vi "burst_config.vi"(8 "error in (no error)":errorcluster, 11 "wf_multi":T1(array[cluster])=[{"device"="waveform_gen", "chan"=1}, {"device"="wf_33500B", "chan"=2}] {"chan" items=["1"=1, "2"=2]}) -> (0 "error out":errorcluster, 1 "cmds":string[](array[string])=["SOUR1:BURS:PHAS 0;\nSOUR1:BURS:MODE GAT;\nSOUR1:BURS:STAT ON;\nTRIG1:SLOP POS;\nTRIG1:DEL 0;\nTRIG1:SOUR EXT;", "SOUR1:BURS:PHAS 0;\nSOUR1:BURS:MODE GAT;\nSOUR1:BURS:STAT ON;\nTRIG1:SLOP POS;\nTRIG1:DEL 0;\nTRIG1:SOUR EXT;"])   [LabVIEW 2017, in "wf.lvlib"]
uses:
  wf.lvlib
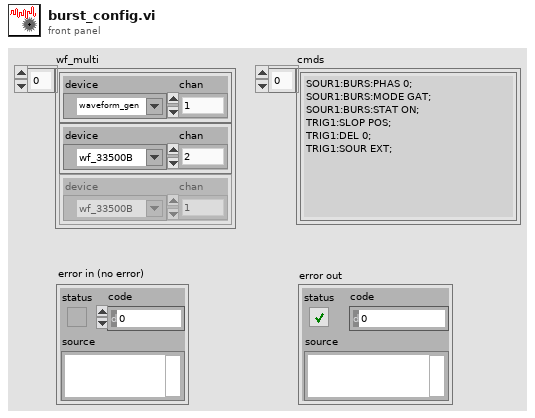
[diagram p1: front panel]
types:
  T1 = cluster{"device":refnum<visa-resource-name>, "chan":i32}[]
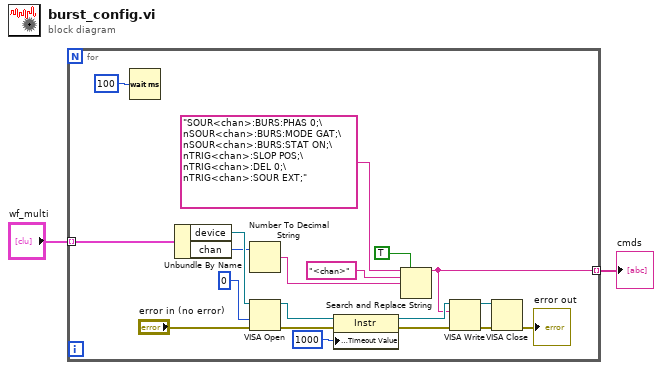
[diagram p0: block diagram]
diagram:
  n1 = for {
    tunnel: "wf_multi" -> [w13] mode=indexing
    tunnel: [w4] -> w2 mode=indexing
    n2 = Wait (ms)(milliseconds to wait=u32 100) -> ()  [unwired: 1 out]
    n3 = Unbundle By Name(w13) -> ("device"=w12:refnum<visa-resource-name>, "chan"=w6:i32)
    n4 = Number To Decimal String(number=w6) -> (decimal integer string=w5:string)  [unwired: 1 in]
    n5 = VISA Open(access mode=u32 0, error in (no error)="error in (no error)", VISA resource name=w12) -> (VISA resource name=w10:refnum<visa-resource-name>, error out=w11:errorcluster)  [unwired: 2 out]
    n6 = property class="Instr"(reference=w10, error in=w11, "General Settings:Timeout Value"=u32 1000) -> (reference out=w15:refnum<visa-resource-name>, error out=w17:errorcluster)
    n7 = Search and Replace String(replace all?=TRUE ("replace all? (F)"), input string="SOUR<chan>:BURS:PHAS 0;\nSOUR<chan>:BURS:MODE GAT;\nSOUR<chan>:BURS:STAT ON;\nTRIG<chan>:SLOP POS;\nTRIG<chan>:DEL 0;\nTRIG<chan>:SOUR EXT;" ("write buffer"), search string="<chan>", replace string=w5) -> (result string=w4:string)  [unwired: 4 in, 3 out]
    n8 = VISA Write(VISA resource name=w15, write buffer=w4, error in (no error)=w17) -> (VISA resource name out=w14:refnum<visa-resource-name>, error out=w16:errorcluster)  [unwired: 1 out]
    n9 = VISA Close(VISA resource name=w14, error in (no error)=w16) -> (error out=→"error out":errorcluster)
  }
  "cmds" <- w2
